vi "Set Ratios.vi"(8 "error in":errorcluster, 9 "Start Index":i32, 10 "PWM Ratios":dbl[](array[numeric]) format="%.3g", 11 "BNT_ULx-MCSV-DOPWM in":refnum<class "BNT_ULx-MCSV-DOPWM.lvclass">) -> (0 "error out":errorcluster, 3 "BNT_ULx-MCSV-DOPWM out":refnum<class "BNT_ULx-MCSV-DOPWM.lvclass">)   [LabVIEW 2020, in "BNT_ULx.lvlib" / "BNT_ULx-MCSV-DOPWM.lvclass"]
doc: "Set pulse width ratios."
uses:
  BNT_ULx-MCSV-DOPWM.lvclass
  BNT_ULx-MCSV-DOPWM.lvclass/BNT_ULx-MCSV-DOPWM.ctl
  CSPP_Core/Classes/CSPP_ProcessVariables/PVConnection/PVConnection.lvclass
  CSPP_Core/Classes/CSPP_ProcessVariables/ProcessVariable/PV.lvclass
  BNT_ULx-MCSV/BNT_ULx-MCSV.lvclass
  C:/User/Brand/LVP/CSPP/CSPP-Template/Packages/BNT_ULx/BNT_ULx-MCSV/BNT_ULx-MCSV/BNT_ULx-MCSV.lvclass
  C:/User/Brand/LVP/CSPP/CSPP-Template/Packages/CSPP_Core/Actors/CSPP_DeviceActor/CSPP_DeviceActor.lvclass
  C:/User/Brand/LVP/CSPP/CSPP-Template/Packages/CSPP_Core/Actors/CSPP_BaseActor/CSPP_BaseActor.lvclass
  C:/Program Files (x86)/National Instruments/LabVIEW 2020/vi.lib/ActorFramework/Actor/Actor.lvclass
  C:/User/Brand/LVP/CSPP/CSPP-Template/Packages/BNT_ULx/BNT_ULx-MCSV/BNT_ULx-MCSV-DOPWM/BNT_ULx-MCSV-DOPWM.lvclass
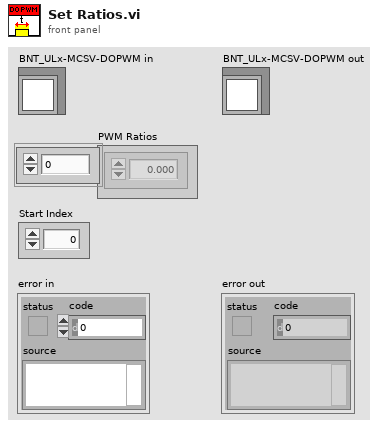
[diagram p1: front panel]
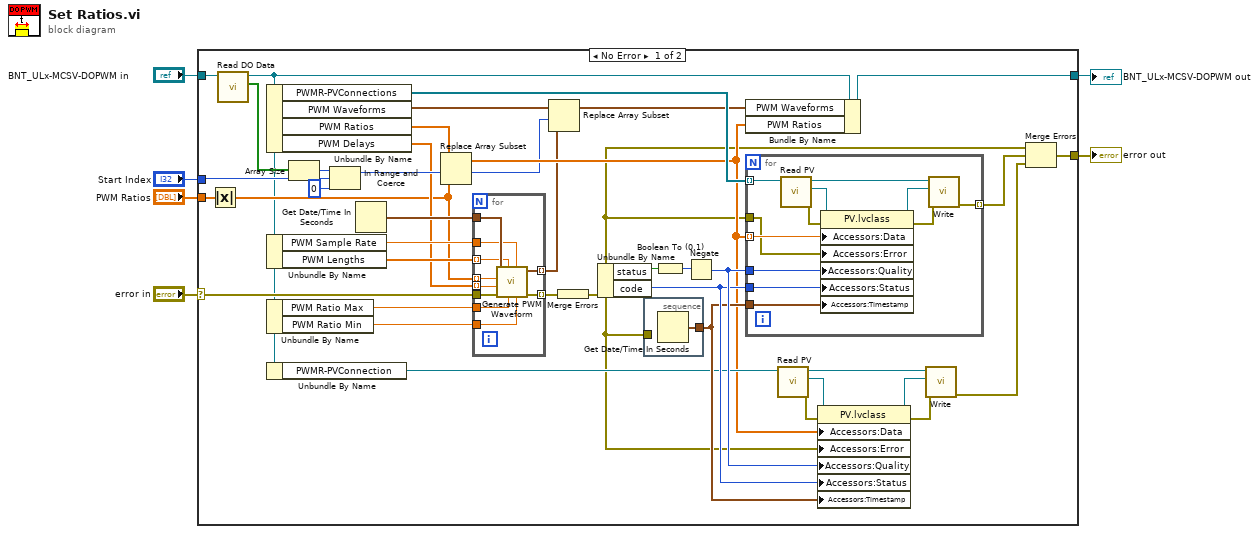
[diagram p0: block diagram]
diagram:
  n1 = case shown="No Error" "error in" {
    selector: "error in" -> [w17 w70]
    tunnel: [w42 w70] -> w2
    tunnel: [w40 w69] -> w1
    tunnel: "BNT_ULx-MCSV-DOPWM in" -> [w8 w69]
    tunnel: "PWM Ratios" -> [w12 _]
    tunnel: "Start Index" -> [w21 _]
    frame No Error {
      n2 = Absolute Value(x=w12) -> (abs(x)=w10:dbl[])
      n3 = call "Read DO Data.vi"("BNT_DAQmx-MCSV in"=w8) -> ("DO Data"=w9:bool[], "BNT_DAQmx-MCSV out"=w7:refnum<class "BNT_ULx-MCSV-DOPWM.lvclass">)  [unwired: 8 in, 1 out]
      n4 = Unbundle By Name(w7) -> ("PWMR-PVConnections"=w41:refnum<class "PVConnection.lvclass">[], "PWM Waveforms"=w28:waveform(dbl)[], "PWM Ratios"=w29:dbl[], "PWM Delays"=w11:dbl[])
      n5 = Unbundle By Name(w7) -> ("PWM Sample Rate"=w16:dbl[unit], "PWM Lengths"=w15:dbl[unit][])
      n6 = Unbundle By Name(w7) -> ("PWM Ratio Max"=w14:dbl, "PWM Ratio Min"=w13:dbl)
      n7 = Unbundle By Name(w7) -> ("PWMR-PVConnection"=w30:refnum<class "PVConnection.lvclass">)
      n8 = Array Size(array=w9) -> (size(s)=w23:i32)
      n9 = In Range and Coerce(upper limit=w23, x=w21, lower limit=0) -> (coerced(x)=w22:i32)  [unwired: 1 out]
      n10 = Get Date/Time In Seconds() -> (seconds since 1Jan1904=w18:timestamp)
      n11 = Replace Array Subset(array=w29, new element=w10, index=w22) -> (w26:dbl[])
      n12 = for {
        tunnel: w18 -> [w52]
        tunnel: [w55] -> w19 mode=indexing
        tunnel: [w54] -> w20 mode=indexing
        tunnel: w16 -> [w46]
        tunnel: w15 -> [w47] mode=indexing
        tunnel: w10 -> [w50] mode=indexing
        tunnel: w14 -> [w49]
        tunnel: w13 -> [w48]
        tunnel: w17 -> [w53]
        tunnel: w11 -> [w51] mode=indexing
        n13 = call "Generate PWM Waveform.vi"("PWM Ratio Min"=w48, "PWM Sample Rate"=w46, "PWM Ratio Max"=w49, "PWM Length"=w47, "error in (no error)"=w53, "PWM Delay"=w51, "PWM Ratio"=w50, "Timestamp"=w52) -> ("error out"=w54:errorcluster, "PWM Waveform"=w55:waveform(dbl))  [unwired: 2 in]
      }
      n14 = Replace Array Subset(array=w28, new element=w19, index=w22) -> (w27:waveform(dbl)[])
      n15 = Merge Errors(w20) -> (w25:errorcluster)
      n16 = Unbundle By Name(w25) -> ("status"=w44:bool, "code"=w33:i32)
      n17 = stacked-sequence {
        tunnel: [w56] -> w32
        tunnel: w25 -> [_]
        frame #0 {
          n18 = Get Date/Time In Seconds() -> (seconds since 1Jan1904=w56:timestamp)
        }
      }
      n19 = Boolean To (0,1)(Boolean=w44) -> (0, 1=w45:i16)
      n20 = Negate(x=w45) -> (-x=w34:i16)
      n21 = Bundle By Name(cluster=w7, "PWM Waveforms"=w27, "PWM Ratios"=w26) -> (w40:refnum<class "BNT_ULx-MCSV-DOPWM.lvclass">)
      n22 = for {
        tunnel: w41 -> [w60] mode=indexing
        tunnel: w26 -> [w68] mode=indexing
        tunnel: w25 -> [w67]
        tunnel: [w64] -> w43 mode=indexing
        tunnel: w34 -> [w63]
        tunnel: w33 -> [w62]
        tunnel: w32 -> [w61]
        n23 = call "Read PV.vi"("PVConnection in"=w60) -> ("error out"=w57:errorcluster, "PV"=w58:refnum<class "PV.lvclass">, "PVConnection out"=w59:refnum<class "PVConnection.lvclass">)  [unwired: 8 in]
        n24 = property class="PV.lvclass"(reference=w58, error in=w57, "Accessors:Data"=w68, "Accessors:Error"=w67, "Accessors:Quality"=w63, "Accessors:Status"=w62, "Accessors:Timestamp"=w61) -> (reference out=w66:refnum<class "PV.lvclass">, error out=w65:errorcluster)
        n25 = call "Write.vi"("error in (no error)"=w65, "PV"=w66, "PVConnection in"=w59) -> ("error out"=w64:errorcluster)  [unwired: 6 in, 2 out]
      }
      n26 = call "Read PV.vi"("PVConnection in"=w30) -> ("error out"=w39:errorcluster, "PV"=w38:refnum<class "PV.lvclass">, "PVConnection out"=w37:refnum<class "PVConnection.lvclass">)  [unwired: 8 in]
      n27 = property class="PV.lvclass"(reference=w38, error in=w39, "Accessors:Data"=w26, "Accessors:Error"=w25, "Accessors:Quality"=w34, "Accessors:Status"=w33, "Accessors:Timestamp"=w32) -> (reference out=w35:refnum<class "PV.lvclass">, error out=w36:errorcluster)
      n28 = call "Write.vi"("error in (no error)"=w36, "PV"=w35, "PVConnection in"=w37) -> ("error out"=w31:errorcluster)  [unwired: 6 in, 2 out]
      n29 = Merge Errors(w25, w43, w31) -> (w42:errorcluster)
    }
    frame Error {
    }
  }
  "error out" <- w2
  "BNT_ULx-MCSV-DOPWM out" <- w1
